vi "SDCP SMF Transmitter and Receiver - Plot Trace File.vi"() -> ()   [LabVIEW 2020]
panel:
  in  "Stop file index":u16
  in  "Start file index":u16
  in  "Start Time (ms)":dbl
  in  "Time axis span (ms)":dbl
  out "Value":dbl
  out "Time (ms)":dbl
  in  "Cursor Plot":string(combo)
  in  "Stop Application":bool
  out "Plot Loaded":bool
  in  "End Parameter Name":string(combo)
  in  "Start Parameter Name":string(combo)
  out "XY Graph":T1(graph)
  in  "Trace File Path":path=path "E:/Projects/System Diagnostics and Control Protocol/SDCP_LabVIEW/temp/Trace Files/TRACE_13_05_2024__23_10_17/0.csv"
  in  "Parameter file path":path=path "E:/Projects/System Diagnostics and Control Protocol/SDCP_LabVIEW/Parameter Files/Motion_Processing.param"
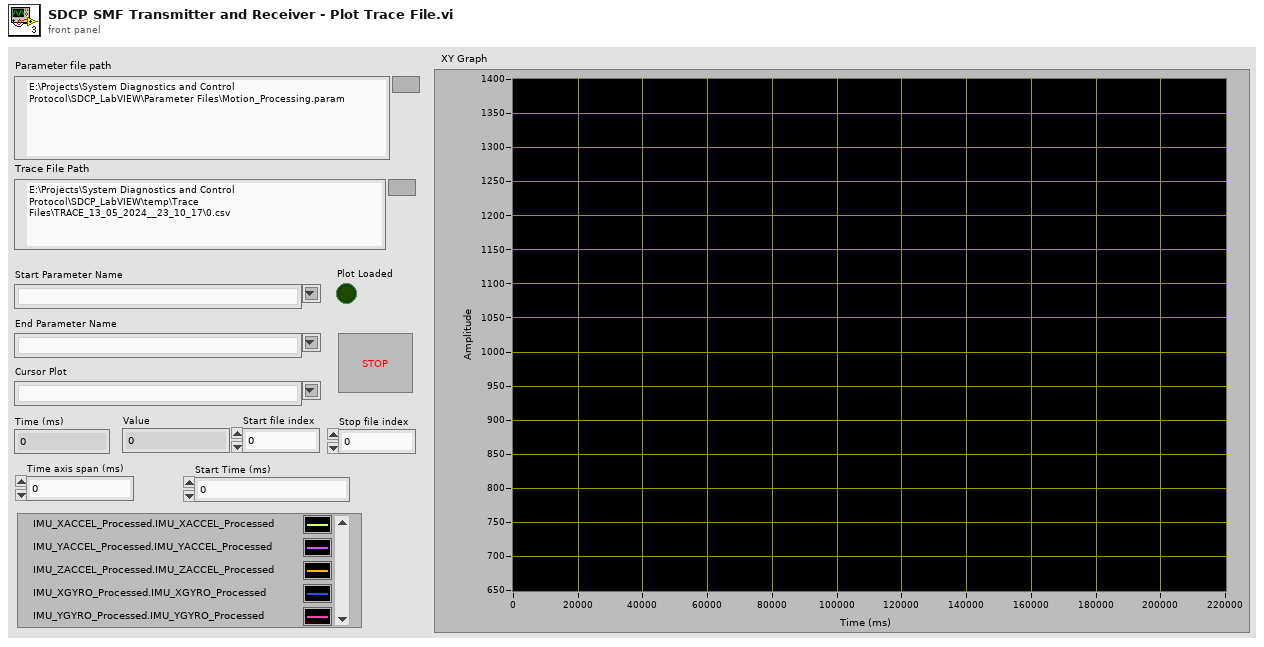
[diagram p1: front panel]
types:
  T1 = cluster{"Plot data":cluster{"X":dbl, "Y":dbl}[]}[]
  T2 = cluster{"Plot data":cluster{"X":dbl, "Y":dbl}[], "Plot name":string}[]
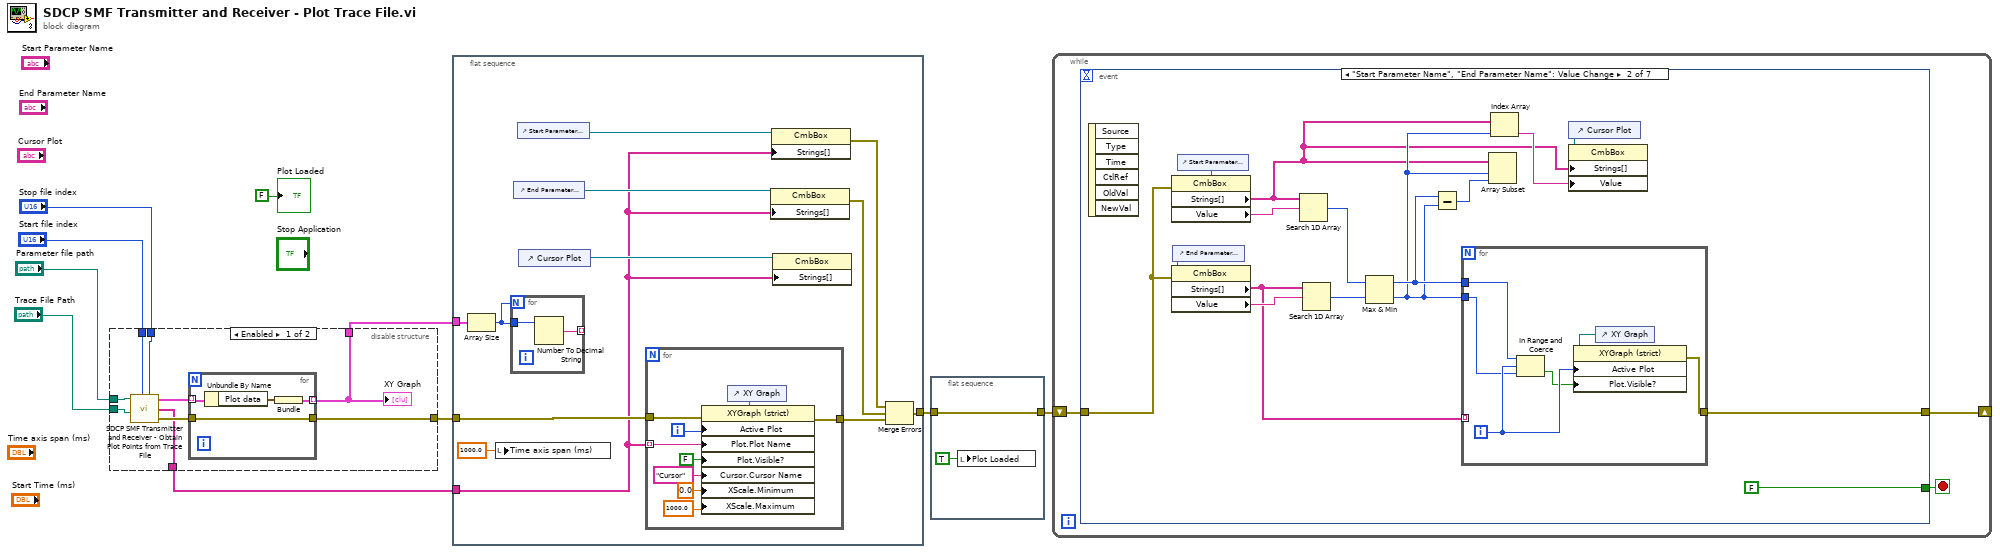
[diagram p0: block diagram]
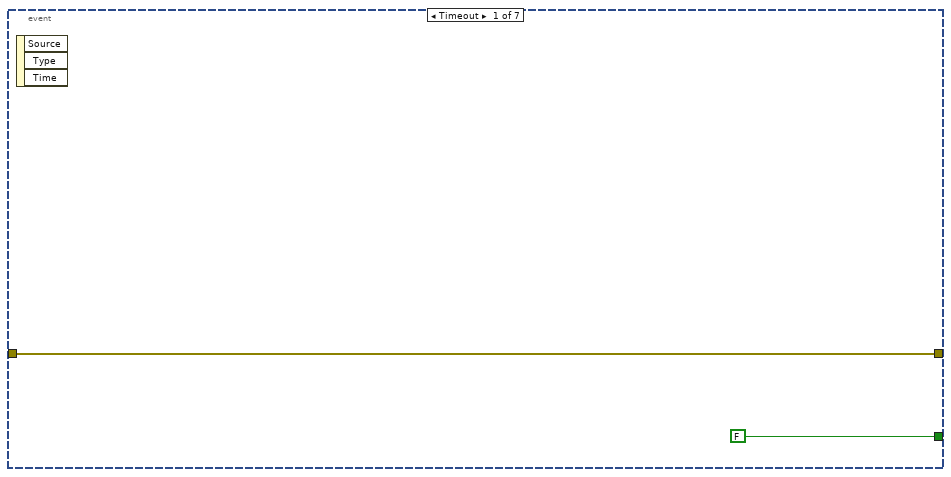
[diagram p2: hidden frame]
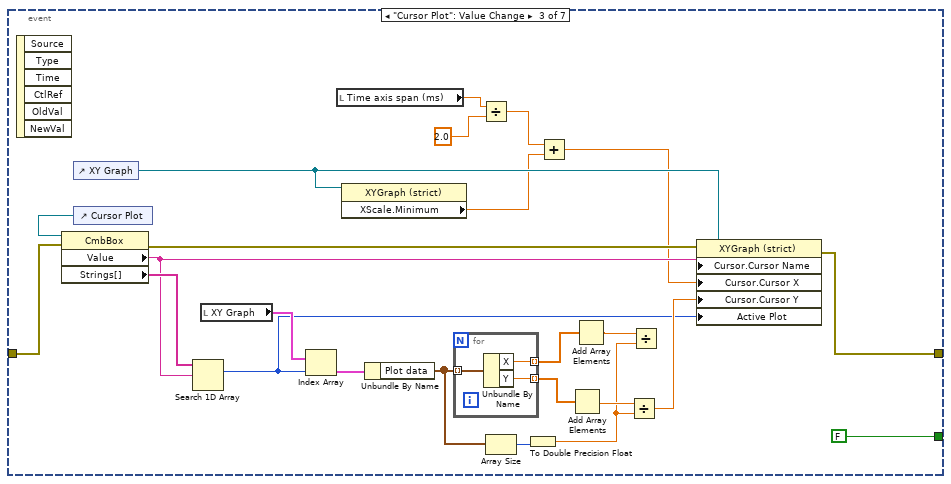
[diagram p3: hidden frame]
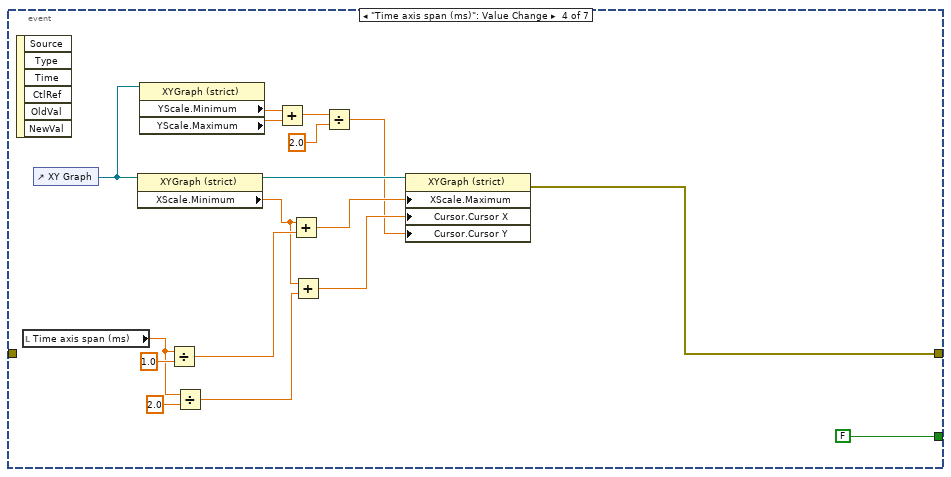
[diagram p4: hidden frame]
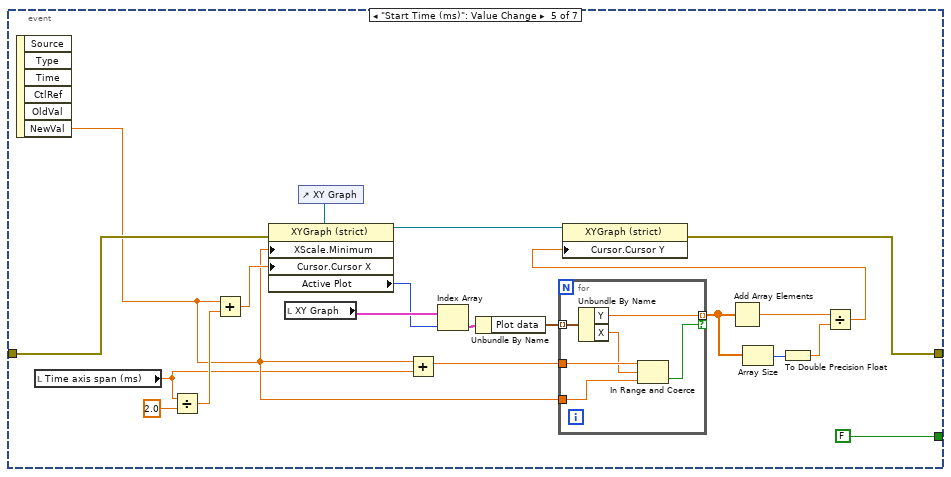
[diagram p5: hidden frame]
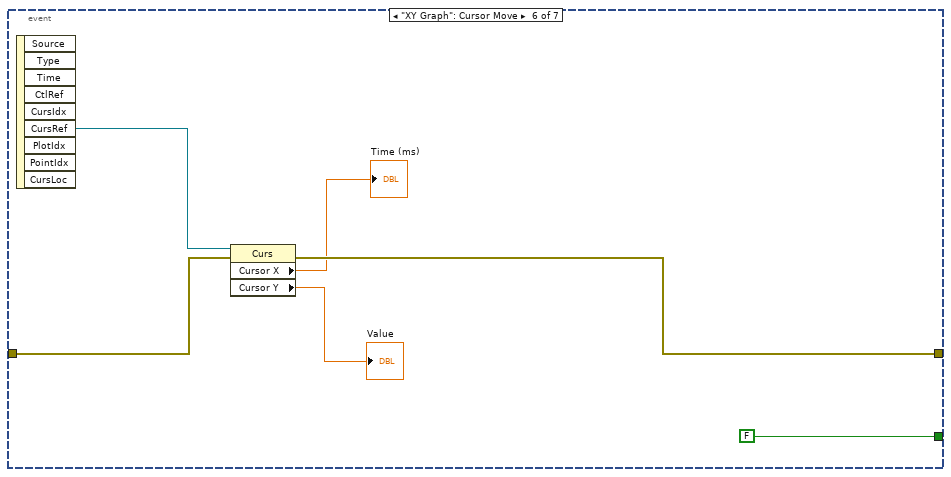
[diagram p6: hidden frame]
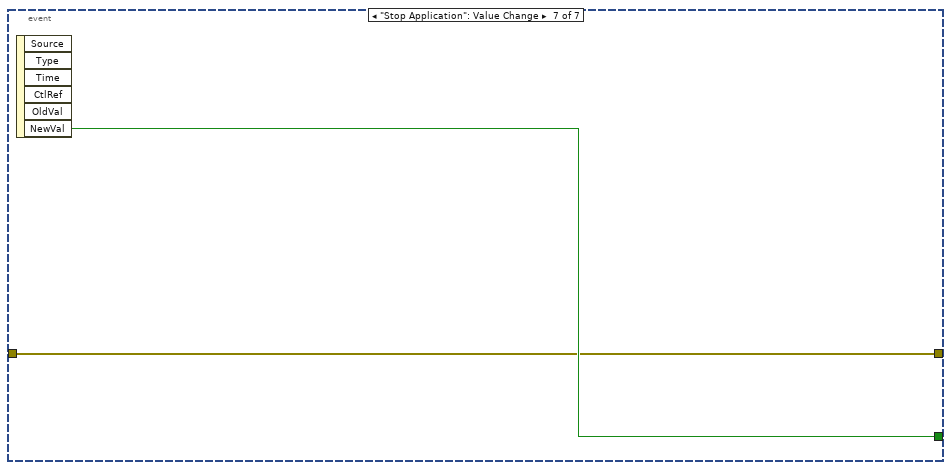
[diagram p7: hidden frame]
diagram:
  n1 = disable-structure shown="Enabled" {
    disable-tunnel: "Parameter file path" -> [w19 _]
    disable-tunnel: "Trace File Path" -> [w18 _]
    disable-tunnel: [w15 _] -> w8
    disable-tunnel: [w14 _] -> w7
    disable-tunnel: [w13 _] -> w6
    disable-tunnel: "Start file index" -> [w12 _]
    disable-tunnel: "Stop file index" -> [w11 _]
    frame Enabled {
      n2 = call "SDCP SMF Transmitter and Receiver - Obtain Plot Points from Trace File.vi"("Stop file index"=w11, "Trace File Path"=w18, "Start file index"=w12, "Parameter file path"=w19) -> ("error out"=w16:errorcluster, "Parameter names"=w14:string[], "Plot details"=w17:T2)  [unwired: 4 in]
      n3 = for {
        tunnel: w17 -> [w23] mode=indexing
        tunnel: [w21] -> w13 mode=indexing
        tunnel: w16 -> [w20]
        tunnel: [w20] -> w15
        n4 = Unbundle By Name(w23) -> ("Plot data"=w22:cluster{"X":dbl, "Y":dbl}[])
        n5 = Bundle("Plot data"=w22) -> (w21:cluster{"Plot data":cluster{"X":dbl, "Y":dbl}[]})  [unwired: 1 in]
      }
      "XY Graph" <- w13
    }
    frame Disabled {
    }
  }
  n6 = flat-sequence {
    tunnel: w8 -> [w35]
    tunnel: w7 -> [w25]
    tunnel: w6 -> [w32]
    tunnel: [w27] -> w5
    frame #0 {
      n7 = Array Size(array=w32) -> (size(s)=w31:i32)
      n8 = local write "Time axis span (ms)"(1000.0 ("Time axis span (ms)")) -> ()
      n9 = for {
        N: w31 -> [_]
        tunnel: w31 -> [w37]
        tunnel: [w36] -> _ mode=indexing
        n10 = Number To Decimal String(number=w37) -> (decimal integer string=w36:string)  [unwired: 1 in]
      }
      n11 = control-ref of="End Parameter Name"() -> (w33:refnum<vi>)
      n12 = control-ref of="Start Parameter Name"() -> (w34:refnum<vi>)
      n13 = control-ref of="Cursor Plot"() -> (w26:refnum<vi>)
      n14 = for {
        tunnel: w35 -> [w46]
        tunnel: w25 -> [w44] mode=indexing
        tunnel: [w41] -> w30
        i -> [w43]
        n15 = control-ref of="XY Graph"() -> (w45:refnum<vi>)
        n16 = property class="XYGraph (strict)"(reference=w45, error in=w46, "Active Plot"=w43, "Plot.Plot Name"=w44, "Plot.Visible?"=FALSE ("Plot.Visible"), "Cursor.Cursor Name"="Cursor", "XScale.Minimum"=0.0 ("X Scale.Range:Minimum"), "XScale.Maximum"=1000.0 ("X Scale.Range:Maximum")) -> (error out=w41:errorcluster)  [unwired: 1 out]
      }
      n17 = property class="CmbBox"(reference=w33, "Strings[]"=w25) -> (error out=w29:errorcluster)  [unwired: 1 in, 1 out]
      n18 = property class="CmbBox"(reference=w34, "Strings[]"=w25) -> (error out=w28:errorcluster)  [unwired: 1 in, 1 out]
      n19 = property class="CmbBox"(reference=w26, "Strings[]"=w25) -> ()  [unwired: 1 in, 2 out]
      n20 = Merge Errors(w28, w29, w30) -> (w27:errorcluster)
    }
  }
  n21 = flat-sequence {
    tunnel: w5 -> [w48]
    tunnel: [w48] -> w4
    frame #0 {
      n22 = local write "Plot Loaded"(TRUE ("Plot Loaded")) -> ()
    }
  }
  n23 = while {
    shift-right: [w49] -> _
    shift-left: w4 -> [w50]
    stop <- w51 stop-if-true
    n24 = event shown="[1] \"Start Parameter Name\", \"End Parameter Name\": Value Change" {
      selector: _ -> [_ _ _ _ _ _ _]
      dyn-events: _ -> [_ _ _ _ _ _ _]
      timeout: _ -> [_ _ _ _ _ _ _]
      tunnel: [FALSE FALSE FALSE ("NewVal") FALSE ("NewVal") FALSE ("NewVal") FALSE ("NewVal") w153] -> w51
      tunnel: w50 -> [w52 w66 w91 _ w137 w150 w152]
      tunnel: [w52 w63 w96 w103 w120 w148 w152] -> w49
      event Timeout {
        n25 = event-data() -> ()  [unwired: 1 in, 3 out]
      }
      event "Start Parameter Name", "End Parameter Name": Value Change {
        n26 = event-data() -> ()  [unwired: 1 in, 6 out]
        n27 = control-ref of="End Parameter Name"() -> (w67:refnum<vi>)
        n28 = property class="CmbBox"(reference=w67, error in=w66) -> ("Strings[]"=w62:string[], "Value"=w64:string)  [unwired: 2 out]
        n29 = control-ref of="Start Parameter Name"() -> (w68:refnum<vi>)
        n30 = property class="CmbBox"(reference=w68, error in=w66) -> ("Strings[]"=w54:string[], "Value"=w65:string)  [unwired: 2 out]
        n31 = Search 1D Array(1D array=w54, element=w65) -> (index of element=w61:i32)  [unwired: 1 in]
        n32 = Search 1D Array(1D array=w62, element=w64) -> (index of element=w60:i32)  [unwired: 1 in]
        n33 = Max & Min(x=w61, y=w60) -> (max(x,y)=w59:i32, min(x,y)=w56:i32)
        n34 = Subtract(x=w59, y=w56) -> (x-y=w58:i32)
        n35 = for {
          tunnel: [w74] -> w63
          tunnel: w62 -> [_] mode=indexing
          tunnel: w59 -> [w73]
          tunnel: w56 -> [w70]
          i -> [w72]
          n36 = In Range and Coerce(upper limit=w73, x=w72, lower limit=w70) -> (In Range?=w71:bool)  [unwired: 1 out]
          n37 = control-ref of="XY Graph"() -> (w75:refnum<vi>)
          n38 = property class="XYGraph (strict)"(reference=w75, "Active Plot"=w72, "Plot.Visible?"=w71) -> (error out=w74:errorcluster)  [unwired: 1 in, 1 out]
        }
        n39 = Array Subset(array=w54, index=w56, length=w58) -> ()  [unwired: 1 out]
        n40 = Index Array(array=w54, index=w56) -> (element=w55:string)
        n41 = control-ref of="Cursor Plot"() -> (w57:refnum<vi>)
        n42 = property class="CmbBox"(reference=w57, "Strings[]"=w54, "Value"=w55) -> ()  [unwired: 1 in, 2 out]
      }
      event "Cursor Plot": Value Change {
        n43 = event-data() -> ()  [unwired: 1 in, 6 out]
        n44 = control-ref of="XY Graph"() -> (w82:refnum<vi>)
        n45 = control-ref of="Cursor Plot"() -> (w98:refnum<vi>)
        n46 = property class="CmbBox"(reference=w98, error in=w91) -> (error out=w97:errorcluster, "Value"=w94:string, "Strings[]"=w95:string[])  [unwired: 1 out]
        n47 = Search 1D Array(1D array=w95, element=w94) -> (index of element=w76:i32)  [unwired: 1 in]
        n48 = local read "XY Graph"() -> (w93:T1)
        n49 = Index Array(array=w93, index=w76) -> (element=w92:cluster{"Plot data":cluster{"X":dbl, "Y":dbl}[]})
        n50 = local read "Time axis span (ms)"() -> (w81:dbl)
        n51 = property class="XYGraph (strict)"(reference=w82) -> ("XScale.Minimum"=w78:dbl)  [unwired: 1 in, 2 out]
        n52 = Unbundle By Name(w92) -> ("Plot data"=w88:cluster{"X":dbl, "Y":dbl}[])
        n53 = for {
          tunnel: w88 -> [w102] mode=indexing
          tunnel: [w101] -> w90 mode=indexing
          tunnel: [w100] -> w89 mode=indexing
          n54 = Unbundle By Name(w102) -> ("X"=w101:dbl, "Y"=w100:dbl)
        }
        n55 = Divide(x=w81, y=2.0) -> (x/y=w79:dbl)
        n56 = Array Size(array=w88) -> (size(s)=w87:i32)
        n57 = To Double Precision Float(number=w87) -> (double precision float=w84:dbl)
        n58 = Add(x=w79, y=w78) -> (x+y=w77:dbl)
        n59 = Add Array Elements(numeric array=w89) -> (sum=w85:dbl)
        n60 = Add Array Elements(numeric array=w90) -> (sum=w86:dbl)
        n61 = Divide(x=w85, y=w84) -> (x/y=w83:dbl)
        n62 = Divide(x=w86, y=w84) -> ()  [unwired: 1 out]
        n63 = property class="XYGraph (strict)"(reference=w82, error in=w97, "Cursor.Cursor Name"=w94, "Cursor.Cursor X"=w77, "Cursor.Cursor Y"=w83, "Active Plot"=w76) -> (error out=w96:errorcluster)  [unwired: 1 out]
      }
      event "Time axis span (ms)": Value Change {
        n64 = event-data() -> ()  [unwired: 1 in, 6 out]
        n65 = local read "Time axis span (ms)"() -> (w114:dbl)
        n66 = control-ref of="XY Graph"() -> (w109:refnum<vi>)
        n67 = property class="XYGraph (strict)"(reference=w109) -> (reference out=w116:refnum<vi>, "XScale.Minimum"=w112:dbl)  [unwired: 1 in, 1 out]
        n68 = property class="XYGraph (strict)"(reference=w109) -> ("YScale.Minimum"=w108:dbl, "YScale.Maximum"=w107:dbl)  [unwired: 1 in, 2 out]
        n69 = Divide(x=w114, y=1.0) -> (x/y=w117:dbl)
        n70 = Divide(x=w114, y=2.0) -> (x/y=w110:dbl)
        n71 = Add(x=w108, y=w107) -> (x+y=w106:dbl)
        n72 = Add(x=w112, y=w117) -> (x+y=w115:dbl)
        n73 = Add(x=w112, y=w110) -> (x+y=w111:dbl)
        n74 = Divide(x=w106, y=2.0) -> (x/y=w104:dbl)
        n75 = property class="XYGraph (strict)"(reference=w116, "XScale.Maximum"=w115, "Cursor.Cursor X"=w111, "Cursor.Cursor Y"=w104) -> (error out=w103:errorcluster)  [unwired: 1 in, 1 out]
      }
      event "Start Time (ms)": Value Change {
        n76 = event-data() -> ("NewVal"=w129:dbl)  [unwired: 1 in, 5 out]
        n77 = local read "Time axis span (ms)"() -> (w128:dbl)
        n78 = Divide(x=w128, y=2.0) -> (x/y=w135:dbl)
        n79 = Add(x=w129, y=w135) -> (x+y=w134:dbl)
        n80 = local read "XY Graph"() -> (w133:T1)
        n81 = control-ref of="XY Graph"() -> (w138:refnum<vi>)
        n82 = property class="XYGraph (strict)"(reference=w138, error in=w137, "XScale.Minimum"=w129, "Cursor.Cursor X"=w134) -> (reference out=w122:refnum<vi>, "Active Plot"=w132:u32)  [unwired: 1 out]
        n83 = Add(x=w129, y=w128) -> (x+y=w127:dbl)
        n84 = Index Array(array=w133, index=w132) -> (element=w131:cluster{"Plot data":cluster{"X":dbl, "Y":dbl}[]})
        n85 = Unbundle By Name(w131) -> ("Plot data"=w130:cluster{"X":dbl, "Y":dbl}[])
        n86 = for {
          tunnel: w130 -> [w145] mode=indexing
          tunnel: w129 -> [w143]
          tunnel: w127 -> [w144]
          tunnel: [w141] -> w126 mode=indexing if=w140
          n87 = Unbundle By Name(w145) -> ("Y"=w141:dbl, "X"=w142:dbl)
          n88 = In Range and Coerce(upper limit=w144, x=w142, lower limit=w143) -> (In Range?=w140:bool)  [unwired: 1 out]
        }
        n89 = Add Array Elements(numeric array=w126) -> (sum=w124:dbl)
        n90 = Array Size(array=w126) -> (size(s)=w125:i32)
        n91 = To Double Precision Float(number=w125) -> (double precision float=w123:dbl)
        n92 = Divide(x=w124, y=w123) -> (x/y=w121:dbl)
        n93 = property class="XYGraph (strict)"(reference=w122, "Cursor.Cursor Y"=w121) -> (error out=w120:errorcluster)  [unwired: 1 in, 1 out]
      }
      event "XY Graph": Cursor Move {
        n94 = event-data() -> ("CursRef"=w151:refnum<vi>)  [unwired: 1 in, 8 out]
        n95 = property class="Curs"(reference=w151, error in=w150) -> (error out=w148:errorcluster, "Cursor X"=→"Time (ms)":dbl, "Cursor Y"=→"Value":dbl)  [unwired: 1 out]
      }
      event "Stop Application": Value Change {
        n96 = event-data() -> ("NewVal"=w153:bool)  [unwired: 1 in, 5 out]
      }
    }
  }
  "Plot Loaded" <- FALSE ("Plot Loaded")
